vi "Memory.Pointer.Copy.Safe.vi"(8 "error in (no error)":errorcluster, 9 "bytes to copy":u64 format="%08x bytes", 10 "dst pointer in":refnum<class "Memory.Pointer.lvclass">, 11 "src pointer in":refnum<class "Memory.Pointer.lvclass">) -> (0 "error out":errorcluster, 1 "bytes to copy":u64 format="%08x bytes", 2 "dst pointer out":refnum<class "Memory.Pointer.lvclass">, 3 "src pointer out":refnum<class "Memory.Pointer.lvclass">)   [LabVIEW 2016, in "Memory Manager.lvlib" / "Memory.Pointer.lvclass"]
doc: "Copies <b>bytes to copy</b> from the memory address pointed to by <b>src pointer</b> to the memory address pointed to by <b>dst pointer</b>.\n\n<b>Note:</b> This VI is <b>safe</b>.\n\nSafe means that this function evaluates that the size parameter of <b>dst pointer</b> is greater than or equal to the size of the requested memory from <b>src pointer</b> to ensure that the destination memory location is an appropriate size before copying data from source to destination. Reading/writing more data to a pointer than it has allocated can corrupt or crash LabVIEW."
uses:
  Memory.Pointer.lvclass
  Memory.Pointer.lvclass/Memory.Pointer.ctl
  Accessors/Get Address.vi
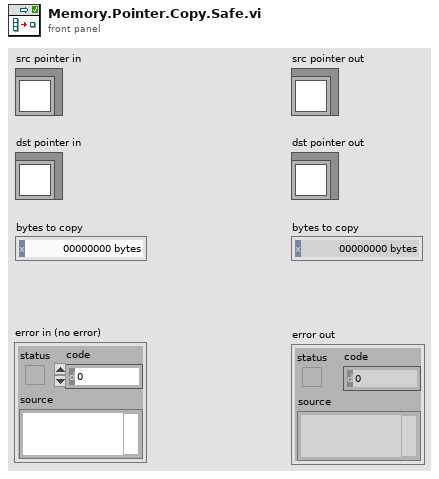
[diagram p1: front panel]
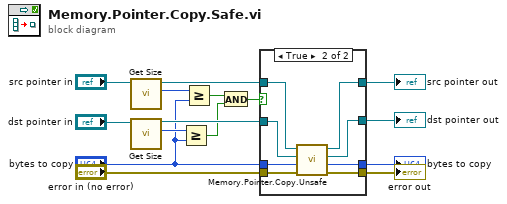
[diagram p0: block diagram]
diagram:
  n1 = call "Get Size.vi"("Pointer in"="src pointer in") -> ("size"=w6:u64, "Pointer out"=w8:refnum<class "Memory.Pointer.lvclass">)  [unwired: 8 in, 1 out]
  n2 = call "Get Size.vi"("Pointer in"="dst pointer in") -> ("size"=w14:u64, "Pointer out"=w10:refnum<class "Memory.Pointer.lvclass">)  [unwired: 8 in, 1 out]
  n3 = Greater Or Equal?(x=w14, y="bytes to copy") -> (x >= y?=w4:bool)
  n4 = Greater Or Equal?(x=w6, y="bytes to copy") -> (x >= y?=w7:bool)
  n5 = And(x=w7, y=w4) -> (x .and. y?=w3:bool)
  n6 = case shown="True" w3 {
    tunnel: [w17 w24] -> w13
    tunnel: "bytes to copy" -> [w17 w25]
    tunnel: w8 -> [w19 w27]
    tunnel: w10 -> [w18 w26]
    tunnel: [w19 w21] -> w12
    tunnel: [w18 w20] -> w11
    tunnel: "error in (no error)" -> [w16 w23]
    tunnel: [w16 w22] -> w1
    frame False {
    }
    frame True {
      n7 = call "Memory.Pointer.Copy.Unsafe.vi"("error in (no error)"=w23, "bytes to copy"=w25, "dst pointer in"=w26, "src pointer in"=w27) -> ("error out"=w22:errorcluster, "bytes to copy"=w24:u64, "dst pointer out"=w20:refnum<class "Memory.Pointer.lvclass">, "src pointer out"=w21:refnum<class "Memory.Pointer.lvclass">)  [unwired: 4 in]
    }
  }
  "error out" <- w1
  "src pointer out" <- w12
  "dst pointer out" <- w11
  "bytes to copy" <- w13
